vi "timer.vi"() -> ()   [LabVIEW 2017]
panel:
  out "迴圈速率(ms)":u32=100
  out "?":i32[][](array[numeric])
  out "最新數據":i32[](array[numeric])
  out "最近10筆紀錄":i32[][](array[numeric])
  out "輸出完整成果":i32[][](array[numeric])
  out "indicator":bool
  in  "Switch":bool
  out "day":dbl(knob) scale=0.0..10.0
  out "hr":dbl(knob) scale=0.0..10.0
  out "min":dbl(knob) scale=0.0..60.0
  out "迴圈執行次數":i32
  in  "stop":bool
  out "s":dbl(knob) scale=0.0..60.0
  # "最新一筆紀錄"
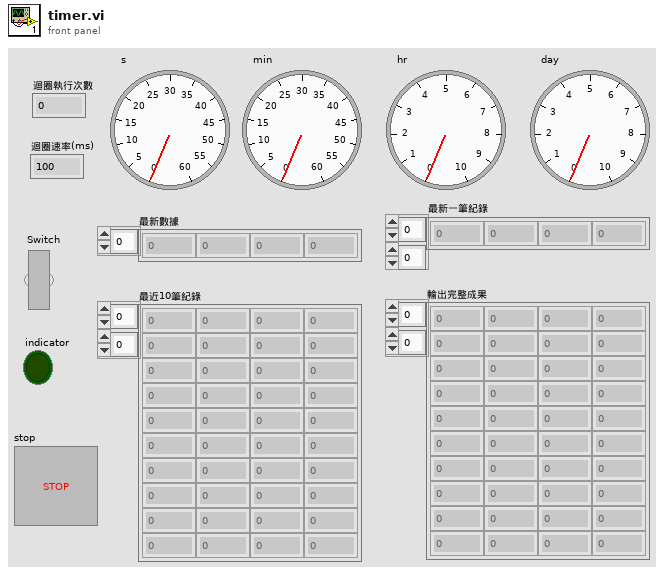
[diagram p1: front panel]
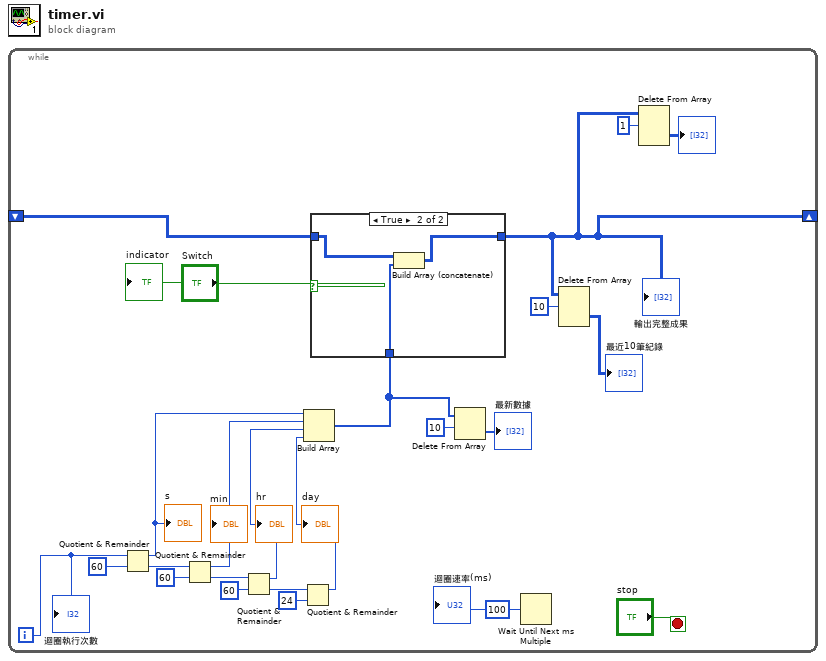
[diagram p0: block diagram]
diagram:
  n1 = while {
    shift-right: [w4] -> _
    shift-left: _ -> [w10]
    i -> [w23]
    stop <- "stop" stop-if-true
    w1 = u32 100 ("millisecond multiple")
    n2 = Quotient & Remainder(x=w23, y=60) -> (x-y*floor(x/y)=w15:i32, floor(x/y)=w21:i32)
    "s" <- w15
    n3 = Quotient & Remainder(x=w21, y=60) -> (x-y*floor(x/y)=w14:i32, floor(x/y)=w19:i32)
    "min" <- w14
    n4 = Quotient & Remainder(x=w19, y=60) -> (x-y*floor(x/y)=w13:i32, floor(x/y)=w17:i32)
    "hr" <- w13
    n5 = Quotient & Remainder(x=w17, y=24) -> (x-y*floor(x/y)=w12:i32)  [unwired: 1 out]
    "day" <- w12
    n6 = Build Array(w15, w14, w13, w12) -> (w6:i32[])
    n7 = case shown="True" "Switch" {
      tunnel: w10 -> [w25 w28]
      tunnel: [w25 w27] -> w4
      tunnel: w6 -> [_ w26]
      frame False {
      }
      frame True {
        n8 = Build Array (concatenate)(w28, w26) -> (w27:i32[][])
      }
    }
    "輸出完整成果" <- w4
    n9 = Delete From Array(array=w6, length=10) -> (deleted portion=→"最新數據":i32[])  [unwired: 1 in, 1 out]
    n10 = Wait Until Next ms Multiple(millisecond multiple=w1) -> ()  [unwired: 1 out]
    n11 = Delete From Array(array=w4, length=10) -> (deleted portion=→"最近10筆紀錄":i32[][])  [unwired: 2 in, 1 out]
    n12 = Delete From Array(array=w4, length=1) -> (deleted portion=→"?":i32[][])  [unwired: 2 in, 1 out]
    "迴圈執行次數" <- w23
    "indicator" <- "Switch"
    "迴圈速率(ms)" <- w1
  }
